vi "Check.vi"(3 "error in (no error)":errorcluster, 4 "StartLotTraveler In":T1, 5 "LotData in":refnum<class "LotData.lvclass">) -> (0 "error out":errorcluster, 1 "StartLotTraveler Out":T1, 2 "LotData out":refnum<class "LotData.lvclass">)   [LabVIEW 2012, in "LotData.lvclass"]
uses:
  Classes/LotData.lvclass
  <vilib>/addons/database/NI_Database_API.lvlib
  <vilib>/addons/database/Connection.llb/Conn Execute.vi
  <vilib>/addons/database/Connection.llb/DB Tools Open Connec (Path).vi
  <vilib>/addons/database/Recordset.llb/Rec Fetch Recordset Data (R).vi
  <vilib>/addons/database/Recordset.llb/Rec Destroy - Connection.vi
  Controls/ProbeStationId.vi
  Controls/StartLotTraveler.ctl
  Controls/MeasurementType.ctl
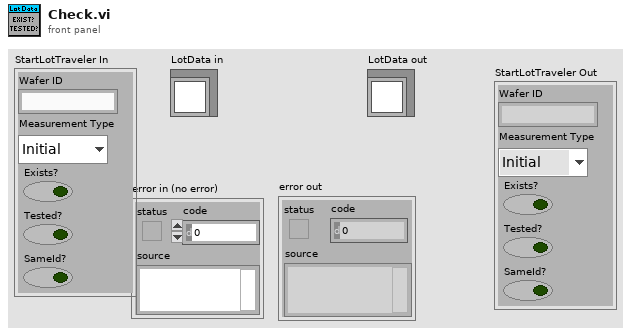
[diagram p1: front panel]
types:
  T1 = typedef "StartLotTraveler.ctl" = cluster{"Wafer ID":string, "Measurement Type":T2, "Exists?":bool, "Tested?":bool, "SameId?":bool}
  T2 = typedef "MeasurementType.ctl" = enum16{"Initial", "Final"}
  T3 = typedef "NI_Database_API.lvlib/Conn ObjectReference.ctl" = refnum<k1>
  T4 = typedef "NI_Database_API.lvlib/Rec ObjectReference.ctl" = refnum<k1>
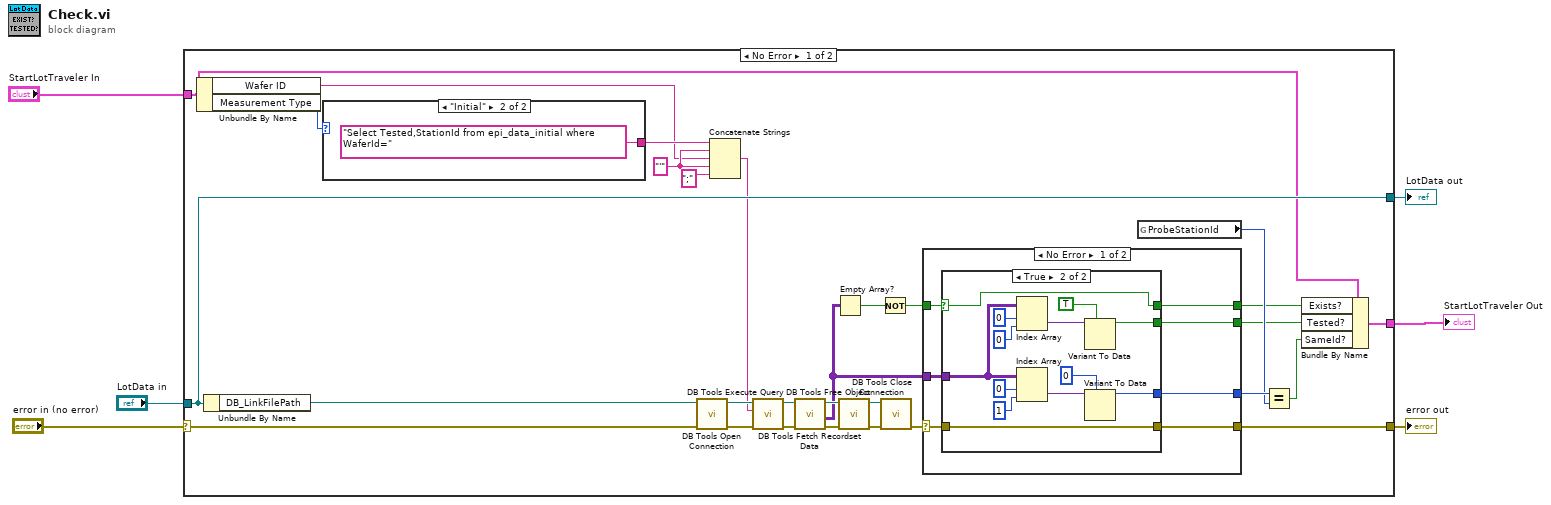
[diagram p0: block diagram]
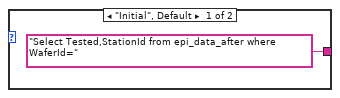
[diagram p2: hidden frame]
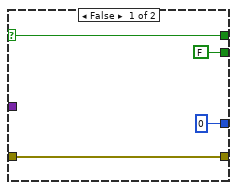
[diagram p3: hidden frame]
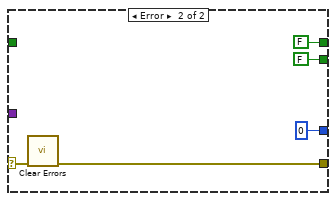
[diagram p4: hidden frame]
diagram:
  n1 = case shown="No Error" "error in (no error)" {
    selector: "error in (no error)" -> [w14 w69]
    tunnel: [w15 w69] -> w6
    tunnel: [w35 w68] -> w5
    tunnel: "LotData in" -> [w35 w68]
    tunnel: "StartLotTraveler In" -> [w11 w67]
    tunnel: [w7 w67] -> w1
    frame No Error {
      w34 = "'" ("string")
      n2 = Unbundle By Name(w11) -> ("Wafer ID"=w12:string, "Measurement Type"=w13:T2)
      n3 = Unbundle By Name(w35) -> ("DB_LinkFilePath"=w20:path)
      n4 = case shown="\"Initial\"" w13 {
        tunnel: ["Select Tested,StationId from epi_data_after where WaferId=" ("string") "Select Tested,StationId from epi_data_initial where WaferId=" ("string")] -> w16
        frame "Initial", Default {
        }
        frame "Initial" {
        }
      }
      n5 = call-poly <vilib>:"DB Tools Open Connection.vi"("error in (no error)"=w14, "connection information"=w20) -> ("error out"=w31:errorcluster, "connection reference"=w32:T3)  [unwired: 6 in]
      n6 = Concatenate Strings(w16, w34, w12, w34, ";" ("string")) -> (w19:string)
      n7 = call-poly <vilib>:"DB Tools Execute Query.vi"("error in (no error)"=w31, "SQL query"=w19, "connection reference"=w32) -> ("error out"=w27:errorcluster, "recordset reference"=w28:T4)  [unwired: 5 in]
      n8 = call-poly <vilib>:"DB Tools Fetch Recordset Data.vi"("error in (no error)"=w27, "recordset reference"=w28) -> ("error out"=w25:errorcluster, "recordset data"=w21:variant[][], "recordset reference out"=w26:T4)  [unwired: 3 in]
      n9 = Empty Array?(array=w21) -> (empty?=w24:bool)
      n10 = call-poly <vilib>:"DB Tools Free Object.vi"("error in (no error)"=w25, "recordset reference"=w26) -> ("error out"=w29:errorcluster, "connection reference"=w30:T3)  [unwired: 8 in]
      n11 = Not(x=w24) -> (.not. x?=w22:bool)
      n12 = call <vilib>:"DB Tools Close Connection.vi"("error in (no error)"=w29, "connection reference"=w30) -> ("error out"=w23:errorcluster)  [unwired: 5 in]
      n13 = case shown="No Error" w23 {
        selector: w23 -> [w41 w66]
        tunnel: w22 -> [w44 _]
        tunnel: [w42 w65] -> w15
        tunnel: w21 -> [w43 _]
        tunnel: [w40 FALSE] -> w8
        tunnel: [w39 FALSE] -> w10
        tunnel: [w38 0] -> w18
        frame No Error {
          n14 = case shown="True" w44 {
            selector: w44 -> [w46 w61]
            tunnel: w43 -> [_ w53]
            tunnel: [w48 w54] -> w42
            tunnel: w41 -> [w48 w54]
            tunnel: [FALSE w50] -> w40
            tunnel: [w46 w61] -> w39
            tunnel: [0 w49] -> w38
            frame False {
            }
            frame True {
              n15 = Index Array(array=w53, index (row)=0, index (col)=0 ("disabled index (col)")) -> (element=w58:variant)
              n16 = Index Array(array=w53, index (row)=0, index (col)=1 ("disabled index (col)")) -> (element=w55:variant)
              n17 = Variant To Data(type=TRUE, Variant=w58) -> (data=w50:bool)  [unwired: 1 in, 1 out]
              n18 = Variant To Data(type=0, Variant=w55) -> (data=w49:i32)  [unwired: 1 in, 1 out]
            }
          }
        }
        frame Error {
          n19 = call <vilib>:"Clear Errors.vi"("error in (no error)"=w66) -> ("error out"=w65:errorcluster)  [unwired: 6 in]
        }
      }
      n20 = global read "ProbeStationId.vi" "ProbeStationId"() -> (w17:i32)
      n21 = Equal?(x=w18, y=w17) -> (x = y?=w9:bool)
      n22 = Bundle By Name(cluster=w11, "Exists?"=w10, "Tested?"=w8, "SameId?"=w9) -> (w7:T1)
    }
    frame Error {
    }
  }
  "error out" <- w6
  "LotData out" <- w5
  "StartLotTraveler Out" <- w1
